vi "OAT D16 P005 filter design.vi"(1 "alias protect in final transition":bool, 2 "stop band attenuation":T1(ring)=enum."72 dB") -> (0 "h":dbl[](array[numeric])=[2.0178168892728076e-05, 3.0449222990159743e-05, -0.00011697435090247272, -0.0003607352535365866, -0.0001405573441925207, 0.000628825715547979, 0.0005550024147680608, -0.001046734425800749, -0.0014382144853253428, 0.0014668990011333413, 0.002971841406916165, -0.0017392183274986231, -0.005389458577176372, 0.0016109040058480007, 0.00894683300382856, -0.0007096267279946278, -0.013948968905601884, -0.0015106916149699228, 0.02084307234675029, 0.0059190595341574465, -0.030497528172617586, -0.014174222720303331, 0.045123533220433616, 0.030522044828413857, -0.07235251427756419, -0.07236836728234927, 0.1617959251667596, 0.4351319949331466, 0.4351319949331466, 0.1617959251667596, -0.07236836728234927, -0.07235251427756419, 0.030522044828413857, 0.045123533220433616, -0.014174222720303331, -0.030497528172617586, 0.0059190595341574465, 0.02084307234675029, -0.0015106916149699228, -0.013948968905601884, -0.0007096267279946278, 0.00894683300382856, 0.0016109040058480007, -0.005389458577176372, -0.0017392183274986231, 0.002971841406916165, 0.0014668990011333413, -0.0014382144853253428, -0.001046734425800749, 0.0005550024147680608, 0.000628825715547979, -0.0001405573441925207, -0.0003607352535365866, -0.00011697435090247272, 3.0449222990159743e-05, 2.0178168892728076e-05] format="%.2f")   [LabVIEW 2017, in "SoundVib_Resampling.lvlib"]
uses:
  <vilib>/addons/Sound and Vibration/Order Analysis/Resample Order Tracking/SoundVib_Resampling.lvlib
panel:
  in  "debug?":bool
  out "inpulse response":dbl[](graph)
  out "frequency response":cluster{i32, dbl, dbl[]}(graph)
  out "pass band":cluster{i32, dbl, dbl[]}(graph)
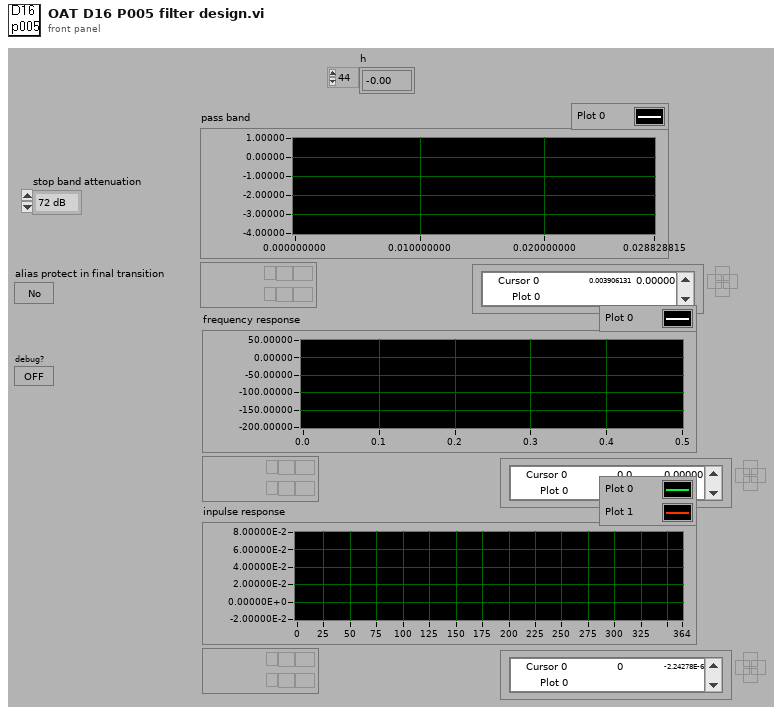
[diagram p1: front panel]
types:
  T1 = enum16{"48 dB", "60 dB", "72 dB", "84 dB", "96 dB", "108 dB", "120 dB"}
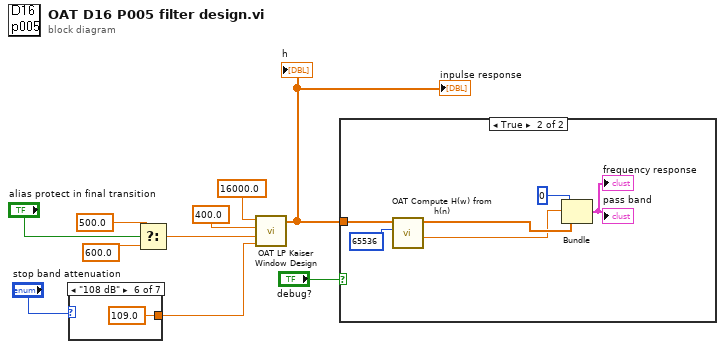
[diagram p0: block diagram]
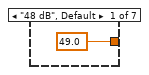
[diagram p2: hidden frame]
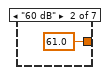
[diagram p3: hidden frame]
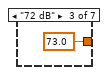
[diagram p4: hidden frame]
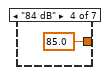
[diagram p5: hidden frame]
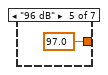
[diagram p6: hidden frame]
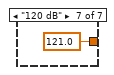
[diagram p7: hidden frame]
diagram:
  n1 = case shown="\"108 dB\"" "stop band attenuation" {
    tunnel: [49.0 61.0 73.0 85.0 97.0 109.0 121.0] -> w1
    frame "48 dB", Default {
    }
    frame "60 dB" {
    }
    frame "72 dB" {
    }
    frame "84 dB" {
    }
    frame "96 dB" {
    }
    frame "108 dB" {
    }
    frame "120 dB" {
    }
  }
  n2 = Select(t=500.0 ("high cutoff freq: fh"), s="alias protect in final transition", f=600.0 ("high cutoff freq: fh")) -> (s? t:f=w7:dbl)
  n3 = call <vilib>:"OAT LP Kaiser Window Design.vi"("A stop [dB]"=w1, "stopband"=w7, "passband"=400.0 ("low cutoff freq: fl"), "fs"=16000.0 ("sampling freq: fs")) -> ("filter coefficients"=w2:dbl[])  [unwired: 5 in, 2 out]
  "h" <- w2
  "inpulse response" <- w2
  n4 = case shown="True" "debug?" {
    tunnel: w2 -> [_ w20]
    frame False {
    }
    frame True {
      n5 = call <vilib>:"OAT Compute H(w) from h(n).vi"("number of frequicies"=65536 ("FFT size"), "h[n]"=w20) -> ("df"=w18:dbl, "amplitude"=w19:dbl[])  [unwired: 7 in, 1 out]
      n6 = Bundle(0, "df"=w18, "amplitude"=w19) -> (→"pass band" →"frequency response":cluster{i32, "df":dbl, "amplitude":dbl[]})  [unwired: 1 in]
    }
  }
